vi "ReadTest_Data.vi"() -> (3 "array":dbl[][](array[numeric]))   [LabVIEW 2020]
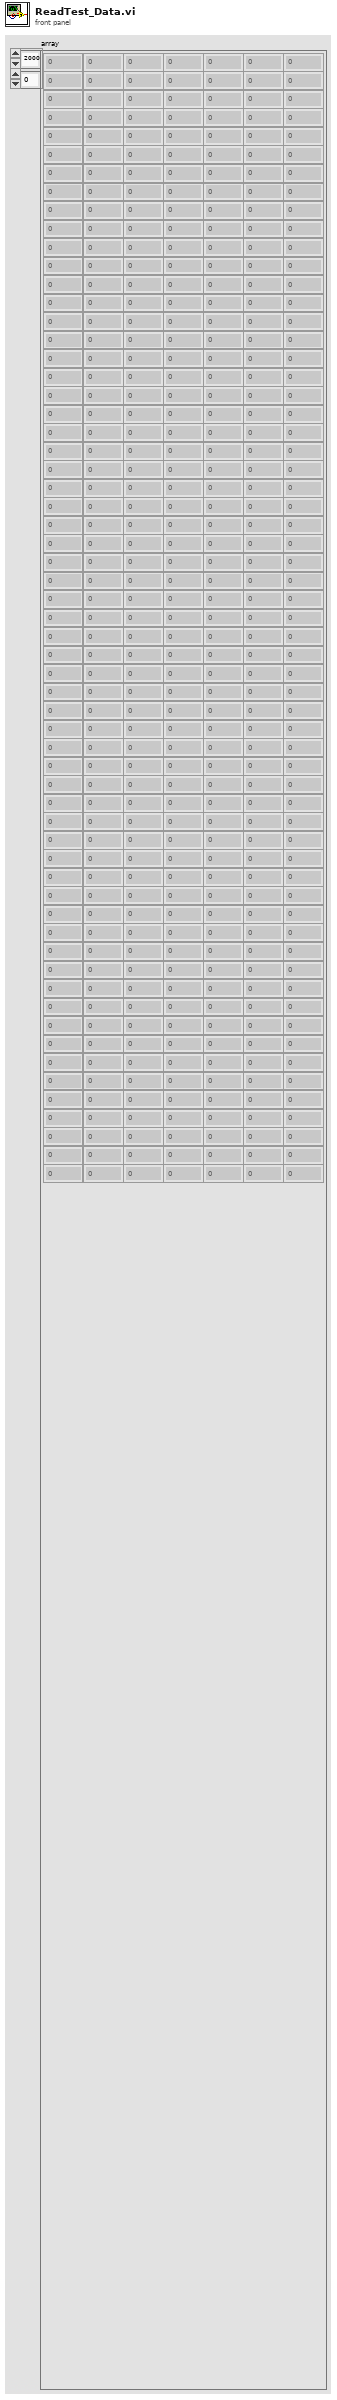
[diagram p1: front panel]
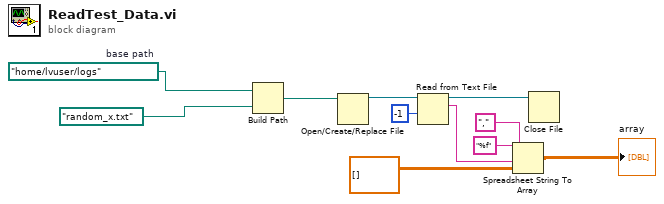
[diagram p0: block diagram]
diagram:
  w9 = path "/home/lvuser/logs"  # base path
  n1 = Build Path(base path=w9, name or relative path=path "random_x.txt") -> (appended path=w10:path)
  n2 = Open/Create/Replace File(file path (use dialog)=w10) -> (refnum out=w8:refnum<file>)  [unwired: 5 in, 2 out]
  n3 = Read from Text File(file (use dialog)=w8, count=-1) -> (refnum out=w4:refnum<file>, text=w6:string)  [unwired: 2 in, 2 out]
  n4 = Spreadsheet String To Array(delimiter (Tab)=",", format string="%f", spreadsheet string=w6, array type (2D Dbl)=sgl[][] []) -> (array=→"array":sgl[][])
  n5 = Close File(refnum=w4) -> ()  [unwired: 1 in, 2 out]
